vi "MasterBatchFileNames.vi"(10 "Raw_Data Folder":path) -> (1 "MasterBatchBackground":path, 2 "MasterBatchAtom":path)   [LabVIEW 2016]
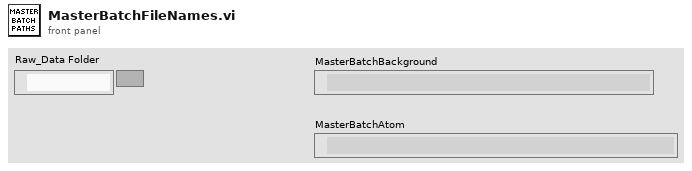
[diagram p1: front panel]
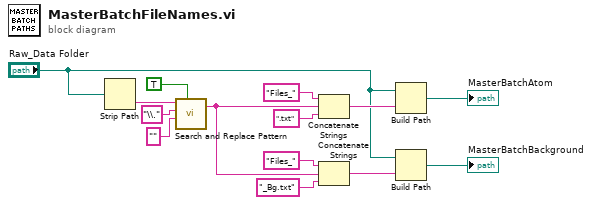
[diagram p0: block diagram]
diagram:
  n1 = Strip Path(path="Raw_Data Folder") -> (name=w14:string)  [unwired: 1 out]
  n2 = call <vilib>:"Search and Replace Pattern.vi"("string"=w14, "regular expression (\"\")"="\\." ("regular expression (\"\")"), "replace string (\"\")"="" ("replace string (\"\")"), "replace all? (F)"=TRUE) -> ("result string"=w4:string)  [unwired: 1 in, 1 out]
  n3 = Concatenate Strings("Files_" ("string"), w4, ".txt" ("string")) -> (w6:string)
  n4 = Concatenate Strings("Files_" ("string"), w4, "_Bg.txt" ("string")) -> (w5:string)
  n5 = Build Path(base path="Raw_Data Folder", name or relative path=w6) -> (appended path=→"MasterBatchAtom":path)
  n6 = Build Path(base path="Raw_Data Folder", name or relative path=w5) -> (appended path=→"MasterBatchBackground":path)
